vi "fgv_gmap-info.vi"(7 "cmd":enum16{"read", "write"}(ring), 8 "error in":errorcluster, 11 "mapinfo":T1) -> (0 "error out":errorcluster, 3 "mapinfo 2":T1)   [LabVIEW 2019]
uses:
  mapinfo.ctl
  C:/Users/WEGO/Documents/GitHub/Patrolrobot/Subvi/Gmap/dll/GMap.NET.WindowsForms.dll
  Patrolrobot/Subvi/Gmap/dll/GMap.NET.WindowsForms.dll
  C:/Users/WEGO/Documents/GitHub/Patrolrobot/Subvi/Gmap/dll/GMap.NET.Core.dll
  Patrolrobot/Subvi/Gmap/dll/GMap.NET.Core.dll
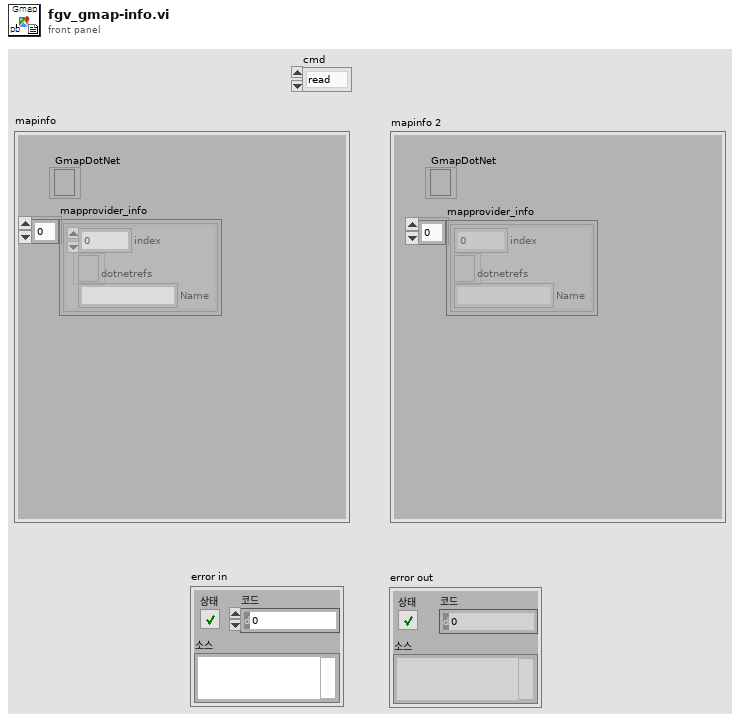
[diagram p1: front panel]
types:
  T1 = typedef "mapinfo.ctl" = cluster{"GmapDotNet":refnum<k24>, "mapprovider_info":cluster{"index":i32, "dotnetrefs":refnum<k24>, "Name":string}[]}
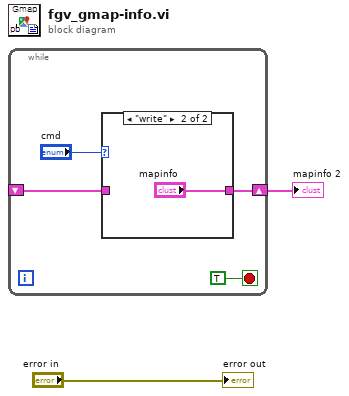
[diagram p0: block diagram]
diagram:
  n1 = while {
    shift-right: [w4] -> w2
    shift-left: _ -> [w3]
    stop <- TRUE stop-if-true
    n2 = case shown="\"write\"" "cmd" {
      tunnel: [w7 "mapinfo"] -> w4
      tunnel: w3 -> [w7 _]
      frame "read", Default {
      }
      frame "write" {
      }
    }
  }
  "mapinfo 2" <- w2
  "error out" <- "error in"
